vi ")Channel.vi"(0 "channel in":T1, 1 "last element in":bool, 2 "This VI":refnum<vi>, 5 "valid":bool=TRUE, 7 "channelOp":T2, 9 "size":i32, 11 "element in":T3, 12 "abort in":bool) -> (3 "last element out":bool, 4 "channel out":T1, 6 "wait":refnum<k4>, 8 "This VI out":refnum<vi>, 10 "count":i32, 13 "retry":bool, 14 "aborted":bool, 15 "element out":T3)   [LabVIEW 2017, in "Stream-t'WPI_EncoderType.ctl'.lvlib"]
uses:
  <extravilib>/ChannelInstances/Stream-t'WPI_EncoderType.ctl'.lvlib
  <vilib>/Rock Robotics/WPI/Encoder/WPI_EncoderType.ctl
  <extravilib>/ChannelInstances/Stream-t'WPI_EncoderType.ctl'/ChannelOp.ctl
  <extravilib>/ChannelInstances/Stream-t'WPI_EncoderType.ctl'/)Channel.ctl
  <extravilib>/ChannelInstances/Stream-t'WPI_EncoderType.ctl'/StreamData.lvclass/StreamData.ctl
  <resource>/ChannelSupport/_ChannelSupport/PipeLogic/PipeLogic.lvclass/PipeLogic.ctl
  <resource>/ChannelSupport/_ChannelSupport/PipeLogic/Status.vi
  <extravilib>/ChannelInstances/Stream-t'WPI_EncoderType.ctl'/GrowArray.vi
  <extravilib>/ChannelInstances/Stream-t'WPI_EncoderType.ctl'/SwapIntoArray.vi
  <resource>/ChannelSupport/_ChannelSupport/PipeLogic/SetSentinel.vi
  <extravilib>/ChannelInstances/Stream-t'WPI_EncoderType.ctl'/SetSize.vi
  <resource>/ChannelSupport/_ChannelSupport/PipeLogic/Init.vi
  <resource>/ChannelSupport/_ChannelSupport/PipeLogic/SetSize.vi
  <resource>/ChannelSupport/_ChannelSupport/SetOccurrence.vi
  <resource>/ChannelSupport/_ChannelSupport/PipeLogic/PipeLogic.lvclass
  <extravilib>/ChannelInstances/Stream-t'WPI_EncoderType.ctl'/StreamData.lvclass
  <resource>/ChannelSupport/_ChannelSupport/_ChannelSupport.lvlib
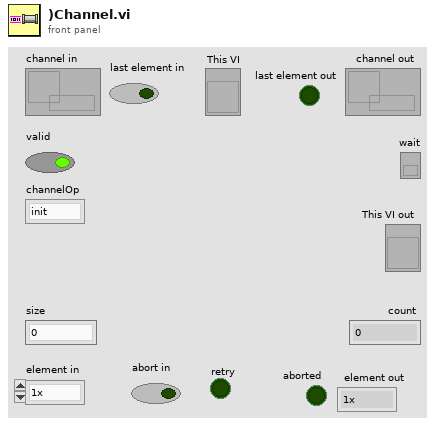
[diagram p1: front panel]
types:
  T1 = typedef "Stream-t'WPI_EncoderType.ctl'.lvlib/)Channel.ctl" = refnum<queue>
  T2 = typedef "Stream-t'WPI_EncoderType.ctl'.lvlib/ChannelOp.ctl" = enum16{"init", "write", "read", "probe"}
  T3 = typedef "WPI_EncoderType.ctl" = enum16{"1x", "2x", "4x"}
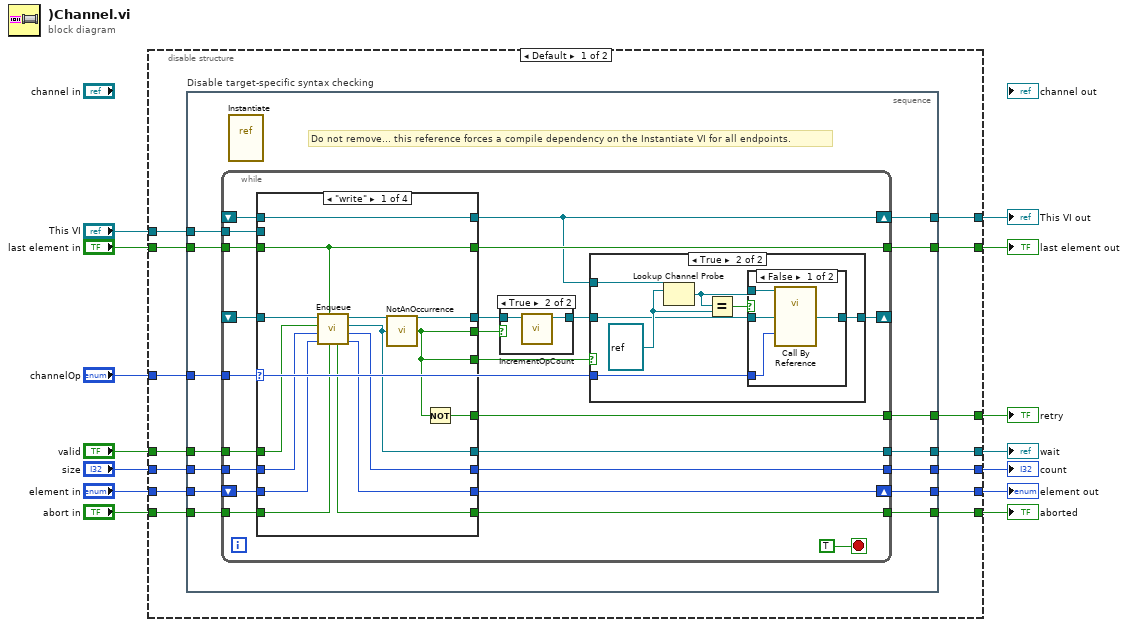
[diagram p0: block diagram]
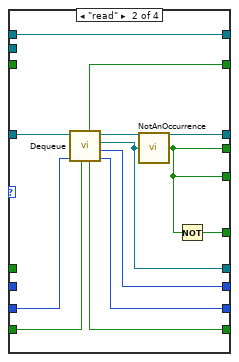
[diagram p5: hidden frame]
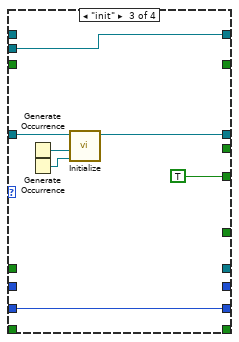
[diagram p6: hidden frame]
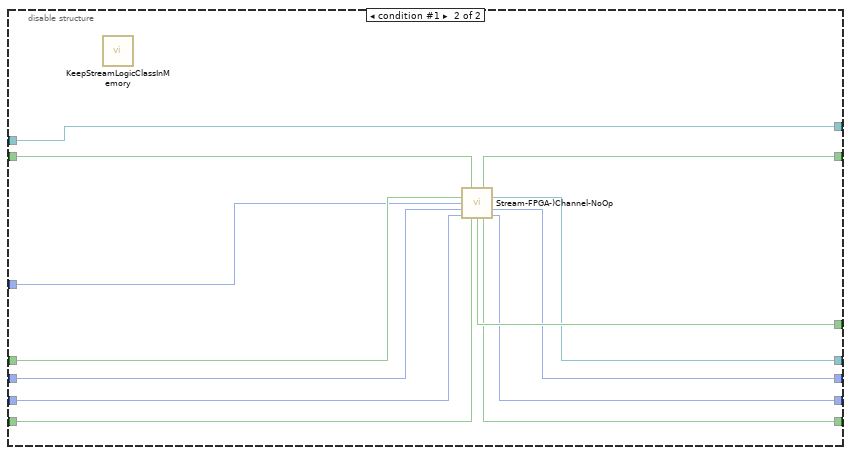
[diagram p8: hidden frame]
diagram:
  n1 = disable-structure "Conditional Disable Structure" shown="Default" {
    disable-tunnel: "element in" -> [w28 w124]
    disable-tunnel: "channelOp" -> [w27 w126]
    disable-tunnel: [w26 w119] -> w12
    disable-tunnel: [w22 w120] -> w11
    disable-tunnel: "size" -> [w25 w125]
    disable-tunnel: "last element in" -> [w24 w129]
    disable-tunnel: [w23 w128] -> w8
    disable-tunnel: [w17 w122] -> w7
    disable-tunnel: "valid" -> [w21 w127]
    disable-tunnel: "abort in" -> [w20 w123]
    disable-tunnel: [w19 w121] -> w4
    disable-tunnel: [w18 w118] -> w3
    disable-tunnel: "This VI" -> [w16 w117]
    disable-tunnel: [w15 w117] -> w1
    frame condition #0 (active) {
      n2 = stacked-sequence "Disable target-specific syntax checking" {
        tunnel: w28 -> [w42]
        tunnel: w27 -> [w41]
        tunnel: [w40] -> w26
        tunnel: w25 -> [w39]
        tunnel: w24 -> [w38]
        tunnel: [w37] -> w23
        tunnel: [w36] -> w22
        tunnel: w21 -> [w35]
        tunnel: w20 -> [w34]
        tunnel: [w33] -> w19
        tunnel: [w32] -> w18
        tunnel: [w31] -> w17
        tunnel: w16 -> [w30]
        tunnel: [w29] -> w15
        frame #0 {
          # "Do not remove... this reference forces a compile dependency on the Instantiate VI for all endpoints."
          n3 = while {
            shift-left: _ -> [w56]
            shift-right: [w45] -> _
            tunnel: w41 -> [w43]
            tunnel: [w62] -> w32
            tunnel: [w61] -> w40
            tunnel: w39 -> [w60]
            tunnel: w38 -> [w59]
            tunnel: [w58] -> w37
            tunnel: w35 -> [w55]
            tunnel: w34 -> [w54]
            tunnel: [w53] -> w33
            tunnel: [w50] -> w31
            tunnel: w30 -> [w49]
            shift-right: [w47] -> w29
            shift-left: _ -> [w48]
            shift-right: [w64] -> w36
            shift-left: w42 -> [w63]
            stop <- TRUE stop-if-true
            n4 = case shown="\"write\"" w43 {
              tunnel: w63 -> [w90 w101 w107 w114]
              tunnel: [w83 w102 w107 w114] -> w64
              tunnel: [w82 w96 _ _] -> w62
              tunnel: [w91 w103 _ _] -> w61
              tunnel: w60 -> [w88 _ _ _]
              tunnel: w59 -> [w92 _ _ _]
              tunnel: [w92 w104 _ _] -> w58
              tunnel: [w93 w105 w112 w116] -> w52
              tunnel: w56 -> [w94 w106 w113 w116]
              tunnel: w55 -> [w89 _ _ _]
              tunnel: w54 -> [w87 w100 _ _]
              tunnel: [w86 w99 _ _] -> w53
              tunnel: [w81 w95 _ _] -> w51
              tunnel: [w85 w98 _ _] -> w50
              tunnel: w49 -> [_ _ w109 _]
              tunnel: [w84 w97 w109 w115] -> w47
              tunnel: w48 -> [w84 w97 _ w115]
              tunnel: [w81 w95 TRUE _] -> w44
              frame "write" {
                n5 = call <resource>:"Enqueue.vi"("abort (F)"=w87, "is last element (F)"=w92, "element in"=w90, "size (0)"=w88, "is valid (T)"=w89, "PipeData in"=w94) -> ("element out"=w83:T3, "count"=w91:i32, "wait"=w82:refnum<k4>, "PipeData out"=w93:refnum<class "StreamData.lvclass">, "aborted?"=w86:bool)  [unwired: 1 in]
                n6 = call <resource>:"NotAnOccurrence.vi"("occurrence refnum"=w82) -> ("not an occurrence?"=w81:bool)
                n7 = Not(x=w81) -> (.not. x?=w85:bool)
              }
              frame "read" {
                n8 = call <resource>:"Dequeue.vi"("abort (F)"=w100, "element in"=w101, "PipeData in"=w106) -> ("element out"=w102:T3, "count"=w103:i32, "wait"=w96:refnum<k4>, "PipeData out"=w105:refnum<class "StreamData.lvclass">, "aborted?"=w99:bool, "last element?"=w104:bool)  [unwired: 3 in]
                n9 = call <resource>:"NotAnOccurrence.vi"("occurrence refnum"=w96) -> ("not an occurrence?"=w95:bool)
                n10 = Not(x=w95) -> (.not. x?=w98:bool)
              }
              frame "init" {
                n11 = Generate Occurrence() -> (w111:refnum<k4>)
                n12 = Generate Occurrence() -> (w110:refnum<k4>)
                n13 = call <extravilib>:"Initialize.vi"("nonempty"=w110, "nonfull"=w111, "PipeData in"=w113) -> ("PipeData out"=w112:refnum<class "StreamData.lvclass">)  [unwired: 8 in]
              }
              frame "probe" {
              }
            }
            n14 = case shown="True" w51 {
              tunnel: w52 -> [w78 w80]
              tunnel: [w78 w79] -> w46
              frame False {
              }
              frame True {
                n15 = call <extravilib>:"IncrementOpCount.vi"("StreamData in"=w80) -> ("StreamData out"=w79:refnum<class "StreamData.lvclass">)  [unwired: 10 in]
              }
            }
            n16 = case shown="True" w44 {
              tunnel: w47 -> [_ w72]
              tunnel: w46 -> [w65 w68]
              tunnel: [w65 w67] -> w45
              tunnel: w43 -> [_ w66]
              frame False {
              }
              frame True {
                w71 = refnum<vi> refnum ("probe type specifier")
                n17 = Lookup Channel Probe(0:w72, 1:w71) -> (9:w69:refnum<vi>)  [unwired: 1 in, 1 out]
                n18 = Equal?(x=w69, y=w71) -> (x = y?=w70:bool)
                n19 = case shown="False" w70 {
                  tunnel: w69 -> [w76 _]
                  tunnel: w68 -> [w75 w77]
                  tunnel: [w74 w77] -> w67
                  tunnel: w66 -> [w73 _]
                  frame False {
                    n20 = call-by-ref "?"(reference=w76, "channelOp"=w73, "PipeData in"=w75) -> ("PipeData out"=w74:refnum<class "StreamData.lvclass">)  [unwired: 2 in, 2 out]
                  }
                  frame True {
                  }
                }
              }
            }
          }
          n21 = vi-ref <extravilib>:"Instantiate.vi"() -> ()  [unwired: 1 out]
        }
      }
    }
    frame condition #1 {
      n22 = call <extravilib>:"KeepStreamLogicClassInMemory.vi"() -> ()  [unwired: 13 in, 3 out]
      n23 = call <extravilib>:"Stream-FPGA-)Channel-NoOp.vi"("sentinel in"=w129, "valid"=w127, "channelOp"=w126, "size"=w125, "element in"=w124, "abort in"=w123) -> ("sentinel out"=w128:bool, "wait"=w118:refnum<k4>, "count"=w119:i32, "retry"=w122:bool, "aborted"=w121:bool, "element out"=w120:T3)  [unwired: 4 in]
    }
  }
  "element out" <- w11
  "count" <- w12
  "last element out" <- w8
  "retry" <- w7
  "aborted" <- w4
  "wait" <- w3
  "This VI out" <- w1
